vi "Calibrate frame period for IGOR.vi"() -> ()   [LabVIEW 2017]
uses:
  <vilib>/gmath/NI_Gmath.lvlib
panel:
  out "Calibrated frame period":dbl
  in  "Measured final trigger position (line number)":string="4.45\n4.450245\n4.4504\n4.4505\n"
  in  "Frame periods empirically entered in IGOR":string="4.45\n4.450245\n4.4504\n4.4505\n"
  in  "Initial trigger position (Line number)":dbl=99.0
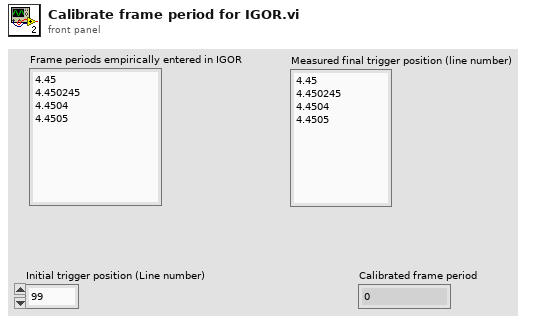
[diagram p1: front panel]
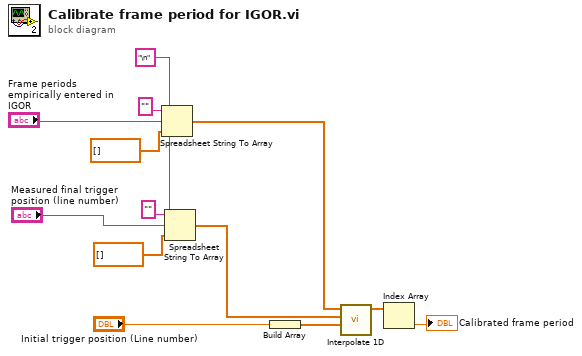
[diagram p0: block diagram]
diagram:
  w7 = "\n" ("delimiter (Tab)")
  n1 = Spreadsheet String To Array(delimiter (Tab)=w7, format string="" ("spreadsheet string"), spreadsheet string="Frame periods empirically entered in IGOR", array type (2D Dbl)=dbl[] [] ("Y")) -> (array=w10:dbl[])
  n2 = Spreadsheet String To Array(delimiter (Tab)=w7, format string="" ("spreadsheet string"), spreadsheet string="Measured final trigger position (line number)", array type (2D Dbl)=dbl[] [] ("Y")) -> (array=w8:dbl[])
  n3 = Build Array("Initial trigger position (Line number)") -> (w13:dbl[])
  n4 = call <vilib>:"Interpolate 1D.vi"("xi"=w13, "X"=w8, "Y"=w10) -> ("yi"=w2:dbl[])  [unwired: 6 in, 2 out]
  n5 = Index Array(array=w2) -> (element=→"Calibrated frame period":dbl)  [unwired: 1 in]
